vi "Prompt for Step--Update State Data.vi"(8 "error in (no error)":errorcluster, 9 "Data":variant, 10 "Argument":string, 11 "Boolean Assertion in":refnum<class "Boolean Assertion.lvclass">) -> (0 "error out":errorcluster, 3 "Boolean Assertion out":refnum<class "Boolean Assertion.lvclass">)   [LabVIEW 2020, in "MacroAssert.lvlib" / "Boolean Assertion.lvclass"]
doc: "Updates the state data within the \"Prompt for Step\" VI."
uses:
  Boolean Assertion.lvclass
  Boolean Assertion Type.ctl
  Assertion Step/Assertion Step.lvclass
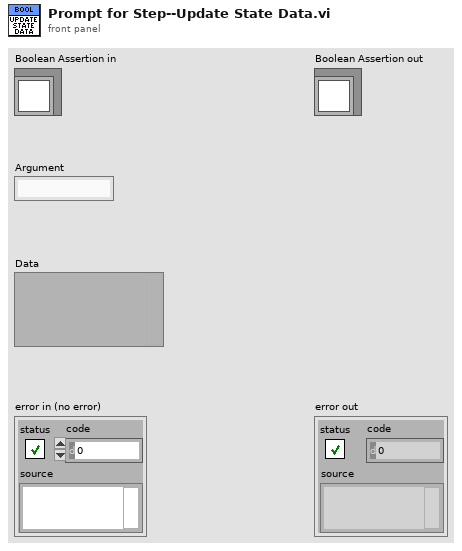
[diagram p1: front panel]
types:
  T1 = typedef "MacroAssert.lvlib/Boolean Assertion.lvclass/Boolean Assertion Type.ctl" = enum16{"Boolean Ctl Value", "Ctl Visible Property", "Ctl is Enabled", "Ctl is Grayed Out", "Ctl Key Focus Property", "Window is in Running Windows", "VI Front Panel is Open"}
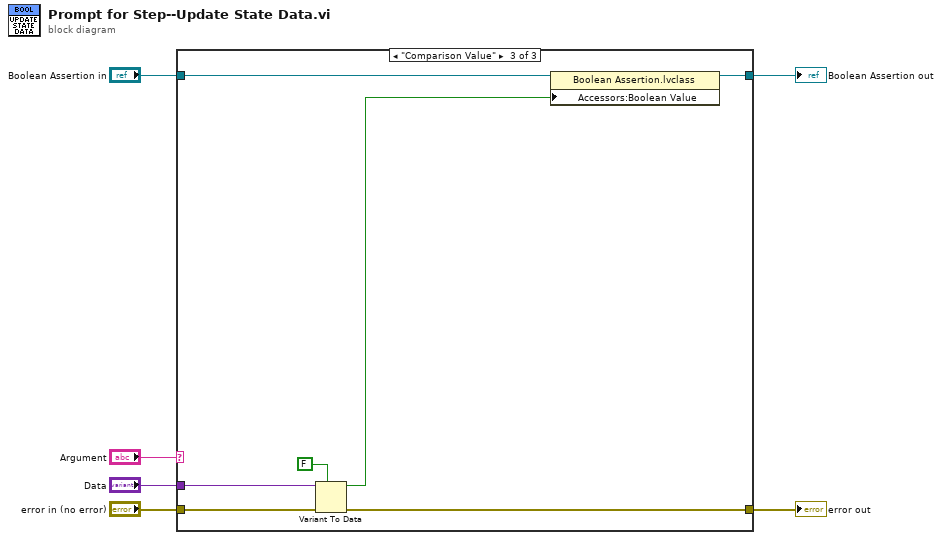
[diagram p0: block diagram]
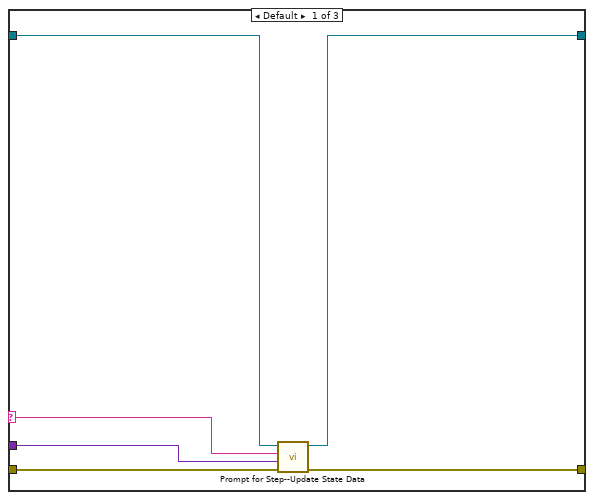
[diagram p2: hidden frame]
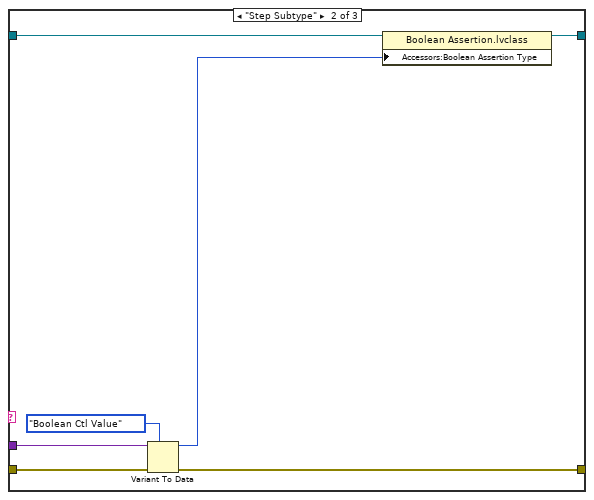
[diagram p3: hidden frame]
diagram:
  n1 = case shown="\"Comparison Value\"" "Argument" {
    selector: "Argument" -> [w9 _ _]
    tunnel: "Boolean Assertion in" -> [w8 w19 w26]
    tunnel: "error in (no error)" -> [w12 w17 w24]
    tunnel: [w7 w18 w25] -> w3
    tunnel: [w11 w16 w23] -> w5
    tunnel: "Data" -> [w10 w14 w22]
    frame Default {
      n2 = call-parent "Prompt for Step--Update State Data.vi"("error in (no error)"=w12, "Data"=w10, "Argument"=w9, "Assertion Step in"=w8) -> ("error out"=w11:errorcluster, "Assertion Step out"=w7:refnum<class "Boolean Assertion.lvclass">)  [unwired: 6 in]
    }
    frame "Step Subtype" {
      n3 = Variant To Data(error in=w17, type=Boolean_Assertion_Type."Boolean Ctl Value" ("Boolean Assertion Type"), Variant=w14) -> (data=w13:T1, error out=w16:errorcluster)
      n4 = property class="Boolean Assertion.lvclass"(reference=w19, "Accessors:Boolean Assertion Type"=w13) -> (reference out=w18:refnum<class "Boolean Assertion.lvclass">)  [unwired: 1 in, 1 out]
    }
    frame "Comparison Value" {
      n5 = Variant To Data(error in=w24, type=FALSE, Variant=w22) -> (data=w21:bool, error out=w23:errorcluster)
      n6 = property class="Boolean Assertion.lvclass"(reference=w26, "Accessors:Boolean Value"=w21) -> (reference out=w25:refnum<class "Boolean Assertion.lvclass">)  [unwired: 1 in, 1 out]
    }
  }
  "error out" <- w5
  "Boolean Assertion out" <- w3
